vi "Read and Update Key.vi"   [LabVIEW 2016, in "User Interface.lvlib" / "User Interface.lvclass"]
uses:
  User Interface.lvclass
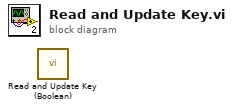
[diagram p0: block diagram]
diagram:
  n1 = call "Read and Update Key (Boolean).vi"() -> ()  [unwired: 9 in, 3 out]
